vi "Final-MurphyE-Sub.vi"(0 "multimeter 1 in":refnum<visa-resource-name>, 1 "Measure? 2 Init Value":bool, 5 "multimeter 2 in":refnum<visa-resource-name>, 7 "function gen in":refnum<visa-resource-name>, 9 "n":i32, 11 "vp-pk to pk array of values":dbl[](array[numeric]), 12 "freq array input":dbl[](array[numeric])) -> (3 "Possible resonant f0 freq\nfor run 2":dbl, 4 "multimeter 1 out":refnum<visa-resource-name>, 6 "multimeter 2 out":refnum<visa-resource-name>, 8 "function gen out":refnum<visa-resource-name>, 10 "freq array output (used)":dbl[](array[numeric]), 13 "vr/vfg rms Cluster for graph":cluster{"freq run 1 list":dbl[], dbl[]}, 14 "Run 2 True Condition Measure Button":bool, 15 "vr/vfg array":dbl[](array[numeric]))   [LabVIEW 2018]
doc: "main while loop for labview program"
uses:
  <vilib>/Analysis/NI_AALBase.lvlib
panel:
  out "Ready For Next Step":bool
  in  "Auto Advance to Next":bool
  in  "Start Taking Measurements?":bool
  out "v across v0 2":dbl
  out "vrms Array":dbl[](array[numeric])
  in  "stop":bool
  out "# Measurements":i32
  out "# Runs":i32
  out "Desired VRMS  (V)":dbl=1.0 min=0.1 max=5.7 step=0.1
  out "freq":dbl
  out "vrms array perfect":dbl[](array[numeric])
  out "Vr0 Vrms":T1(graph)
  out "vfg":dbl
  out "vfg array":dbl[](array[numeric])
  out "Vfg Vrms":T1(graph)
  out "Transfer Function vr0/vfg Vrms":T1(graph)
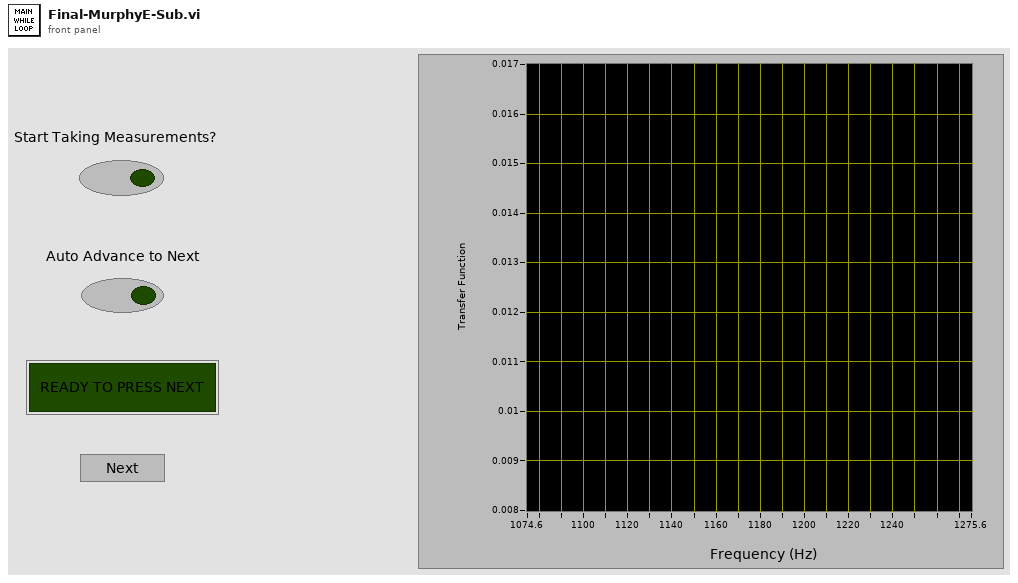
[diagram p1: front panel]
types:
  T1 = cluster{"Ramp Pattern":dbl[], "vrms array":dbl[]}
  T2 = cluster{"freq array input":dbl[], "measured vrms array":dbl[]}
  T3 = cluster{"freq array input":dbl[], "vrms across fg":dbl[]}
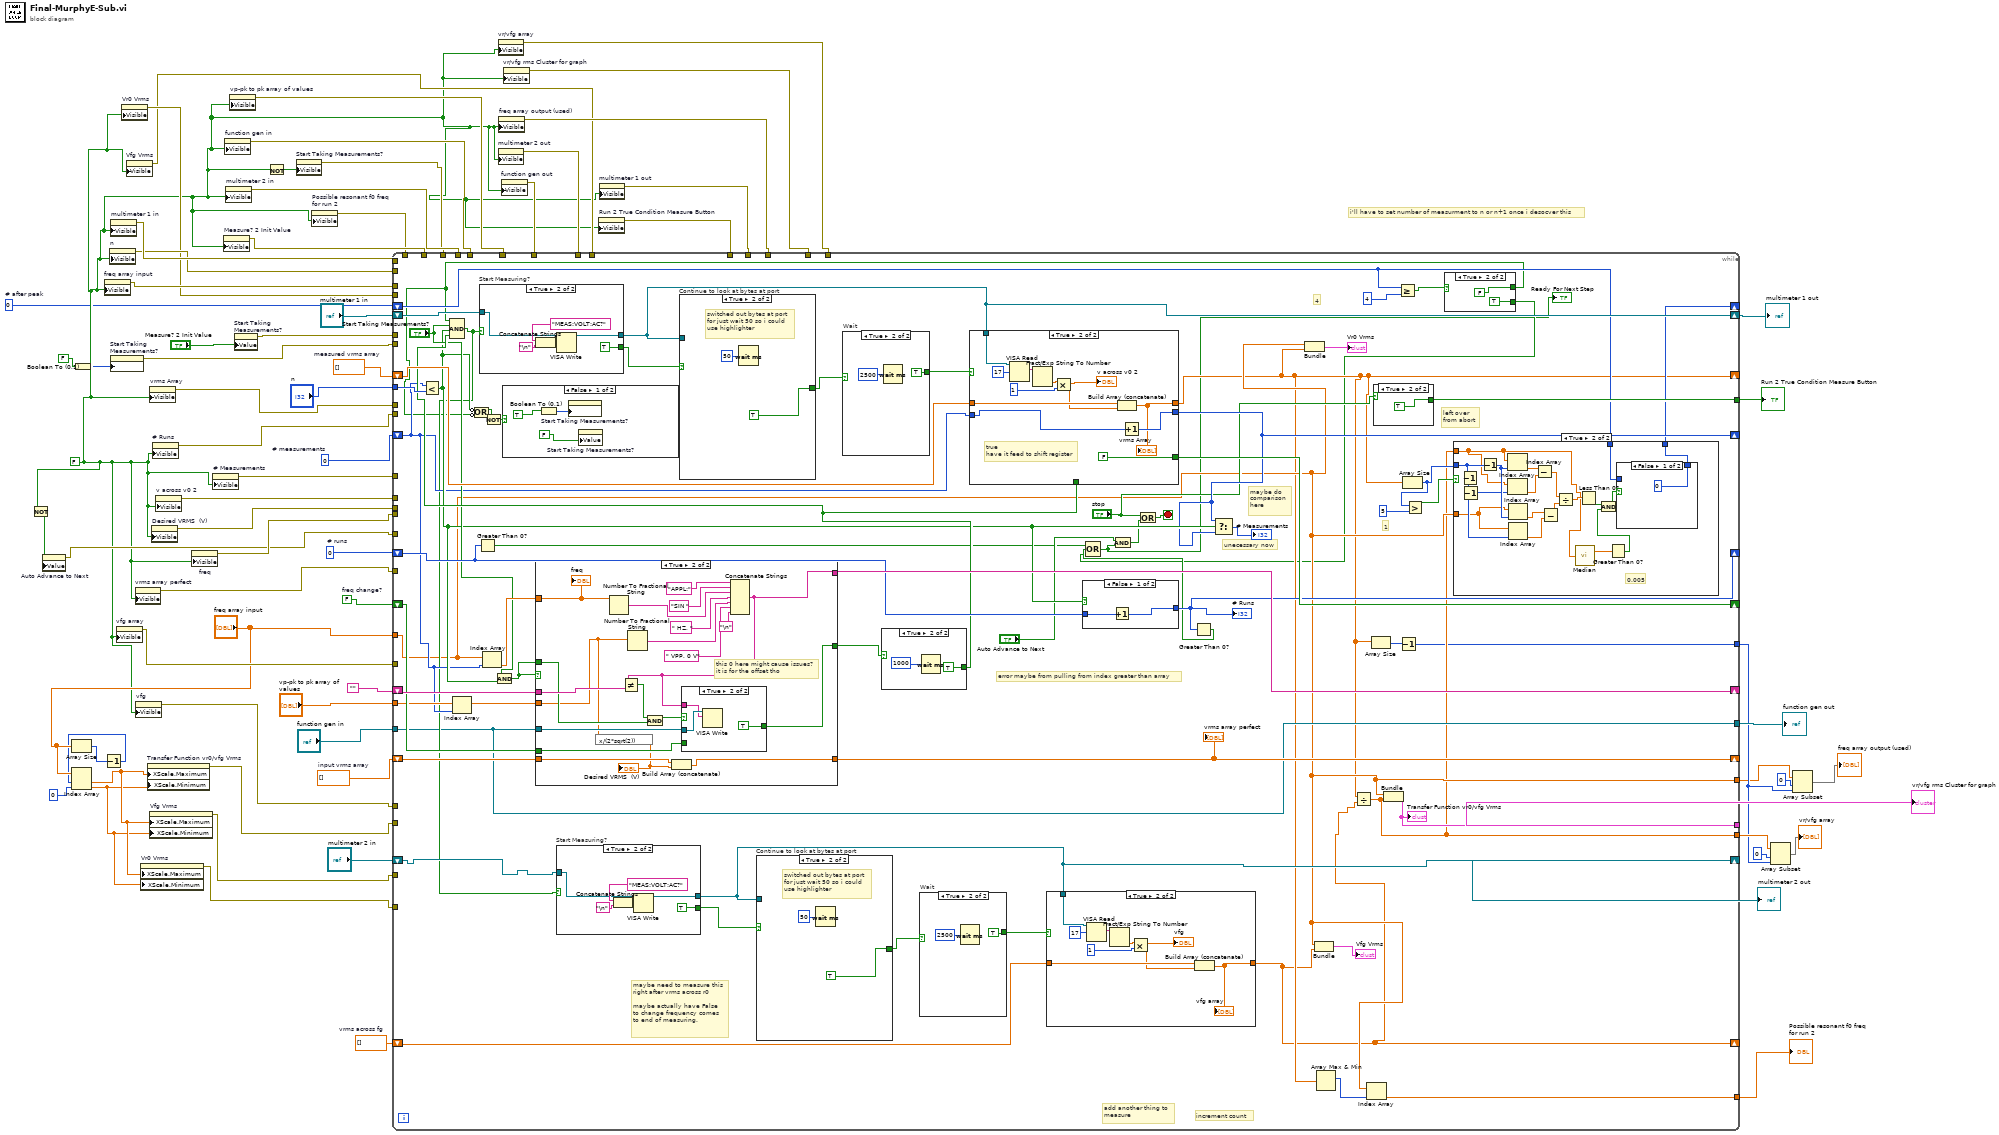
[diagram p0: block diagram]
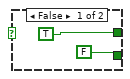
[diagram p2: hidden frame]
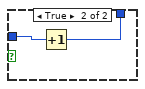
[diagram p4: hidden frame]
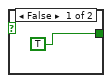
[diagram p5: hidden frame]
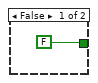
[diagram p7: hidden frame]
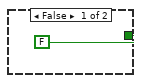
[diagram p8: hidden frame]
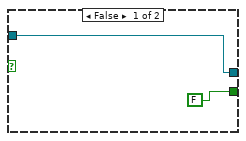
[diagram p9: hidden frame]
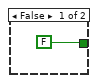
[diagram p16: hidden frame]
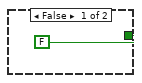
[diagram p17: hidden frame]
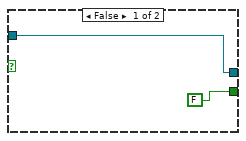
[diagram p18: hidden frame]
diagram:
  w9 = 0  # # after peak
  w68 = 0  # # measurements
  w13 = FALSE
  w60 = dbl[] []  # vrms across fg
  w62 = dbl[] []  # input vrms array
  w66 = FALSE  # freq change?
  w67 = 0  # # runs
  w70 = dbl[] []  # measured vrms array
  # "i'll have to set number of measurment to n or n+1 once i desocver this"
  n1 = Not(x=w13) -> (.not. x?=w8:bool)
  n2 = property on="Auto Advance to Next" class="Bool (strict)"("Value"=w8) -> (error out=w14:errorcluster)  [unwired: 2 in, 1 out]
  n3 = Array Size(array="freq array input") -> (size(s)=w43:i32)
  n4 = Boolean To (0,1)(Boolean=FALSE) -> (0, 1=w10:i16)
  n5 = property on="freq array input" class="Arr (strict)"("Visible"=w13) -> (error out=w20:errorcluster)  [unwired: 2 in, 1 out]
  n6 = Decrement(x=w43) -> (x-1=w42:i32)
  n7 = Index Array(array="freq array input", index #1=w42, index #2=0 ("index")) -> (element #1=w40:dbl, element #2=w39:dbl)
  n8 = property on="n" class="DigNum (strict)"("Visible"=w13) -> (error out=w21:errorcluster)  [unwired: 2 in, 1 out]
  n9 = property on="multimeter 1 in" class="VISAName"("Visible"=w13) -> (error out=w22:errorcluster)  [unwired: 2 in, 1 out]
  n10 = property on="Start Taking Measurements?" class="Bool (strict)"("DisabledEnum"=w10) -> (error out=w12:errorcluster)  [unwired: 2 in, 1 out]
  n11 = property on="vfg array" class="Arr (strict)"("Visible"=w13) -> (error out=w53:errorcluster)  [unwired: 2 in, 1 out]
  n12 = property on="Vr0 Vrms" class="XYGraph (strict)"("Visible"=w13) -> (error out=w16:errorcluster)  [unwired: 2 in, 1 out]
  n13 = property on="Vfg Vrms" class="XYGraph (strict)"("Visible"=w13) -> (error out=w15:errorcluster)  [unwired: 2 in, 1 out]
  n14 = property on="vrms array perfect" class="Arr (strict)"("Visible"=w13) -> (error out=w56:errorcluster)  [unwired: 2 in, 1 out]
  n15 = property on="vfg" class="DigNum (strict)"("Visible"=w13) -> (error out=w52:errorcluster)  [unwired: 2 in, 1 out]
  n16 = property on="Vr0 Vrms" class="XYGraph (strict)"("XScale.Maximum"=w40, "XScale.Minimum"=w39) -> (error out=w36:errorcluster)  [unwired: 2 in, 1 out]
  n17 = property on="Transfer Function vr0/vfg Vrms" class="XYGraph (strict)"("XScale.Maximum"=w40, "XScale.Minimum"=w39) -> (error out=w38:errorcluster)  [unwired: 2 in, 1 out]
  n18 = property on="vrms Array" class="Arr (strict)"("Visible"=w13) -> (error out=w54:errorcluster)  [unwired: 2 in, 1 out]
  n19 = property on="Vfg Vrms" class="XYGraph (strict)"("XScale.Maximum"=w40, "XScale.Minimum"=w39) -> (error out=w37:errorcluster)  [unwired: 2 in, 1 out]
  n20 = property on="Desired VRMS  (V)" class="DigNum (strict)"("Visible"=w13) -> (error out=w58:errorcluster)  [unwired: 2 in, 1 out]
  n21 = property on="# Runs" class="DigNum (strict)"("Visible"=w13) -> (error out=w55:errorcluster)  [unwired: 2 in, 1 out]
  n22 = property on="v across v0 2" class="DigNum (strict)"("Visible"=w13) -> (error out=w59:errorcluster)  [unwired: 2 in, 1 out]
  n23 = property on="freq" class="DigNum (strict)"("Visible"=w13) -> (error out=w57:errorcluster)  [unwired: 2 in, 1 out]
  n24 = property on="# Measurements" class="DigNum (strict)"("Visible"=w13) -> (error out=w45:errorcluster)  [unwired: 2 in, 1 out]
  n25 = property on="Measure? 2 Init Value" class="Bool (strict)"("Visible"=w13) -> (error out=w23:errorcluster)  [unwired: 2 in, 1 out]
  n26 = property on="function gen in" class="VISAName"("Visible"=w13) -> (error out=w25:errorcluster)  [unwired: 2 in, 1 out]
  n27 = property on="multimeter 2 in" class="VISAName"("Visible"=w13) -> (error out=w24:errorcluster)  [unwired: 2 in, 1 out]
  n28 = property on="vp-pk to pk array of values" class="Arr (strict)"("Visible"=w13) -> (error out=w26:errorcluster)  [unwired: 2 in, 1 out]
  n29 = property on="Start Taking Measurements?" class="Bool (strict)"("Value"="Measure? 2 Init Value") -> (error out=w35:errorcluster)  [unwired: 2 in, 1 out]
  n30 = Not(x=w13) -> (.not. x?=w17:bool)
  n31 = property on="Start Taking Measurements?" class="Bool (strict)"("Visible"=w17) -> (error out=w18:errorcluster)  [unwired: 2 in, 1 out]
  n32 = property on="Possible resonant f0 freq\nfor run 2" class="DigNum (strict)"("Visible"=w13) -> (error out=w19:errorcluster)  [unwired: 2 in, 1 out]
  n33 = property on="vr/vfg array" class="Arr (strict)"("Visible"=w13) -> (error out=w33:errorcluster)  [unwired: 2 in, 1 out]
  n34 = property on="multimeter 2 out" class="VISAName"("Visible"=w13) -> (error out=w27:errorcluster)  [unwired: 2 in, 1 out]
  n35 = property on="freq array output (used)" class="Arr (strict)"("Visible"=w13) -> (error out=w31:errorcluster)  [unwired: 2 in, 1 out]
  n36 = property on="function gen out" class="VISAName"("Visible"=w13) -> (error out=w28:errorcluster)  [unwired: 2 in, 1 out]
  n37 = property on="vr/vfg rms Cluster for graph" class="Clust (strict)"("Visible"=w13) -> (error out=w32:errorcluster)  [unwired: 2 in, 1 out]
  n38 = property on="Run 2 True Condition Measure Button" class="Bool (strict)"("Visible"=w13) -> (error out=w30:errorcluster)  [unwired: 2 in, 1 out]
  n39 = property on="multimeter 1 out" class="VISAName"("Visible"=w13) -> (error out=w29:errorcluster)  [unwired: 2 in, 1 out]
  n40 = while {
    shift-right: [w132] -> w46
    shift-left: "multimeter 1 in" -> [w131]
    shift-right: [w109] -> _
    shift-left: w68 -> [w113]
    shift-right: [w77] -> _
    shift-left: w70 -> [w130]
    tunnel: "n" -> [w129]
    shift-right: [w119] -> _
    shift-left: w67 -> [w122]
    tunnel: "freq array input" -> [w86]
    tunnel: "function gen in" -> [w99]
    shift-right: [w126] -> _
    shift-left: "" -> [w127]
    shift-right: [w123] -> _
    shift-left: w66 -> [w124]
    tunnel: "vp-pk to pk array of values" -> [w115]
    shift-right: [w111] -> _
    shift-left: w62 -> [w112]
    shift-right: [w104] -> w49
    shift-left: "multimeter 2 in" -> [w105]
    shift-right: [w75] -> _
    shift-left: w60 -> [w103]
    tunnel: [w99] -> w48
    tunnel: [w98] -> w47
    tunnel: [w97] -> w50
    tunnel: w59 -> [_]
    tunnel: w58 -> [_]
    tunnel: w57 -> [_]
    tunnel: w56 -> [_]
    tunnel: w55 -> [_]
    tunnel: w54 -> [_]
    tunnel: w53 -> [_]
    tunnel: w52 -> [_]
    tunnel: [w86] -> w2
    tunnel: [w85] -> w6
    tunnel: [w96] -> w51
    tunnel: w45 -> [_]
    tunnel: w38 -> [_]
    tunnel: w37 -> [_]
    tunnel: w36 -> [_]
    tunnel: w35 -> [_]
    tunnel: w33 -> [_]
    tunnel: w32 -> [_]
    tunnel: w31 -> [_]
    tunnel: w30 -> [_]
    tunnel: w29 -> [_]
    tunnel: w28 -> [_]
    tunnel: w27 -> [_]
    tunnel: w26 -> [_]
    tunnel: w25 -> [_]
    tunnel: w24 -> [_]
    tunnel: w23 -> [_]
    tunnel: w22 -> [_]
    tunnel: w21 -> [_]
    tunnel: w20 -> [_]
    tunnel: w19 -> [_]
    tunnel: w18 -> [_]
    tunnel: w16 -> [_]
    tunnel: w15 -> [_]
    tunnel: w14 -> [_]
    tunnel: w12 -> [_]
    shift-right: [w84] -> _
    shift-left: w9 -> [w83]
    tunnel: [w74] -> w4
    stop <- w95 stop-if-true
    # "1"
    # "4"
    # "increment count"
    # "add another thing to\nmeasure"
    # "left over\nfrom abort"
    # "maybe need to measure this\nright after vrms across r0\n\nmaybe actually have False\nto change frequency comes\nto end of measuring."
    # "unecessary now"
    # "maybe do\ncomparison\nhere"
    # "error maybe from pulling from index greater than array"
    n41 = Less?(x=w113, y=w129) -> (x < y?=w117:bool)
    n42 = Index Array(array=w115, index=w113) -> (element=w114:dbl)
    n43 = Greater Than 0?(x=w122) -> (x > 0?=w90:bool)
    n44 = Index Array(array=w86, index=w113) -> (element=w125:dbl)
    n45 = Compound Arithmetic op=AND("Start Taking Measurements?", w117) -> (w116:bool)
    n46 = case shown="True" w116 {
      tunnel: w99 -> [_ w205]
      tunnel: w127 -> [w193 w204]
      tunnel: [w193 w203] -> w126
      tunnel: w125 -> [_ w202]
      tunnel: w116 -> [_ w200]
      tunnel: w124 -> [w192 w199]
      tunnel: [w192 w198] -> w121
      tunnel: w114 -> [_ w197]
      tunnel: w112 -> [w191 w196]
      tunnel: [w191 w194] -> w111
      frame False {
      }
      frame True {
        # "this 0 here might cause issues?\nit is for the offset tho"
        n47 = expression code="x/(2*sqrt(2))"(w197) -> (w195:dbl)
        "Desired VRMS  (V)" <- w195
        n48 = Number To Fractional String(number=w202) -> (F-format string=w211:string)  [unwired: 3 in]
        n49 = Number To Fractional String(number=w197) -> (F-format string=w209:string)  [unwired: 3 in]
        n50 = Build Array (concatenate)(w196, w195) -> (w194:dbl[])
        n51 = Concatenate Strings("APPL:", "SIN ", w211, " HZ, ", w209, " VPP, 0 V", "\n") -> (w203:string)
        n52 = Not Equal?(x=w203, y=w204) -> (x != y?=w206:bool)
        n53 = Compound Arithmetic op=AND(w206, w200) -> (w201:bool)
        n54 = case shown="True" w201 {
          tunnel: w203 -> [_ w216]
          tunnel: w205 -> [_ w217]
          tunnel: [w214 TRUE] -> w198
          tunnel: w199 -> [w214 _]
          frame False {
          }
          frame True {
            n55 = VISA Write(VISA resource name=w217, write buffer=w216) -> ()  [unwired: 1 in, 3 out]
          }
        }
        "freq" <- w202
      }
    }
    "vrms array perfect" <- w111
    n56 = case shown="True" w121 {
      selector: w121 -> [w188 _]
      tunnel: [w188 TRUE] -> w120
      frame False {
      }
      frame True {
        n57 = Wait (ms)(milliseconds to wait=u32 1000) -> ()  [unwired: 1 out]
      }
    }
    n58 = case shown="False" w117 {
      tunnel: w122 -> [w219 w220]
      tunnel: [w218 w220] -> w119
      frame False {
        n59 = Increment(x=w219) -> (x+1=w218:i32)
      }
      frame True {
      }
    }
    "# Runs" <- w119
    n60 = Greater Than 0?(x=w119) -> (x > 0?=w93:bool)
    n61 = case shown="True" "stop" {
      tunnel: [TRUE TRUE] -> w98
      frame False {
      }
      frame True {
      }
    }
    n62 = Greater Or Equal?(x=w83, y=4) -> (x >= y?=w81:bool)
    n63 = case shown="True" w81 {
      tunnel: [TRUE FALSE] -> w79
      tunnel: [FALSE TRUE] -> w73
      frame False {
      }
      frame True {
      }
    }
    n64 = Compound Arithmetic op=AND(w79, "Start Taking Measurements?", w117, w120) -> (w102:bool)
    n65 = Compound Arithmetic op=OR(invert w117, invert w79) -> (w80:bool)
    n66 = case "Start Measuring?" shown="True" w102 {
      tunnel: [FALSE TRUE] -> w135
      tunnel: [w244 w247] -> w132
      tunnel: w131 -> [w244 w246]
      frame False {
      }
      frame True {
        n67 = Concatenate Strings("MEAS:VOLT:AC?", "\n") -> (w250:string)
        n68 = VISA Write(VISA resource name=w246, write buffer=w250) -> (VISA resource name out=w247:refnum<visa-resource-name>)  [unwired: 1 in, 2 out]
      }
    }
    n69 = Not(x=w80) -> (.not. x?=w78:bool)
    n70 = case shown="False" w78 {
      frame False {
        n71 = Boolean To (0,1)(Boolean=TRUE) -> (0, 1=w221:i16)
        n72 = property on="Start Taking Measurements?" class="Bool (strict)"("DisabledEnum"=w221) -> ()  [unwired: 2 in, 2 out]
        n73 = property on="Start Taking Measurements?" class="Bool (strict)"("Value"=FALSE) -> ()  [unwired: 2 in, 2 out]
      }
      frame True {
      }
    }
    n74 = case "Start Measuring?" shown="True" w102 {
      tunnel: [FALSE TRUE] -> w108
      tunnel: [w180 w183] -> w104
      tunnel: w105 -> [w180 w182]
      frame False {
      }
      frame True {
        n75 = Concatenate Strings("MEAS:VOLT:AC?", "\n") -> (w186:string)
        n76 = VISA Write(VISA resource name=w182, write buffer=w186) -> (VISA resource name out=w183:refnum<visa-resource-name>)  [unwired: 1 in, 2 out]
      }
    }
    n77 = case "Continue to look at bytes at port" shown="True" w135 {
      tunnel: w132 -> [_ _]
      tunnel: [FALSE TRUE] -> w134
      frame False {
      }
      frame True {
        # "switched out bytes at port\nfor just wait 50 so i could\nuse highlighter"
        n78 = Wait (ms)(milliseconds to wait=u32 50) -> ()  [unwired: 1 out]
      }
    }
    n79 = case "Continue to look at bytes at port" shown="True" w108 {
      tunnel: w104 -> [_ _]
      tunnel: [FALSE TRUE] -> w107
      frame False {
      }
      frame True {
        # "switched out bytes at port\nfor just wait 50 so i could\nuse highlighter"
        n80 = Wait (ms)(milliseconds to wait=u32 50) -> ()  [unwired: 1 out]
      }
    }
    n81 = case "Wait" shown="True" w134 {
      tunnel: [FALSE TRUE] -> w133
      frame False {
      }
      frame True {
        n82 = Wait (ms)(milliseconds to wait=u32 2500) -> ()  [unwired: 1 out]
      }
    }
    n83 = case "Wait" shown="True" w107 {
      tunnel: [FALSE TRUE] -> w106
      frame False {
      }
      frame True {
        n84 = Wait (ms)(milliseconds to wait=u32 2500) -> ()  [unwired: 1 out]
      }
    }
    n85 = case shown="True" w133 {
      tunnel: w132 -> [_ w233]
      tunnel: w113 -> [w226 w229]
      tunnel: [w226 w231] -> w109
      tunnel: w130 -> [w225 w232]
      tunnel: [w225 w230] -> w77
      tunnel: [w224 FALSE] -> w123
      tunnel: w120 -> [w224 _]
      frame False {
      }
      frame True {
        # "true\nhave it feed to shift register"
        n86 = VISA Read(VISA resource name=w233, byte count=17) -> (read buffer=w237:string)  [unwired: 1 in, 3 out]
        n87 = Fract/Exp String To Number(string=w237) -> (number=w234:dbl)  [unwired: 3 in, 1 out]
        n88 = Multiply(x=w234, y=1) -> (x*y=w227:dbl)
        "v across v0 2" <- w227
        n89 = Build Array (concatenate)(w232, w227) -> (w230:dbl[])
        "vrms Array" <- w230
        n90 = Increment(x=w229) -> (x+1=w231:i32)
      }
    }
    n91 = case shown="True" w106 {
      tunnel: w104 -> [_ w169]
      tunnel: w103 -> [w165 w168]
      tunnel: [w165 w166] -> w75
      frame False {
      }
      frame True {
        n92 = VISA Read(VISA resource name=w169, byte count=17) -> (read buffer=w173:string)  [unwired: 1 in, 3 out]
        n93 = Fract/Exp String To Number(string=w173) -> (number=w170:dbl)  [unwired: 3 in, 1 out]
        n94 = Multiply(x=w170, y=1) -> (x*y=w167:dbl)
        "vfg" <- w167
        n95 = Build Array (concatenate)(w168, w167) -> (w166:dbl[])
        "vfg array" <- w166
      }
    }
    n96 = Compound Arithmetic op=OR(w90, w93, w73) -> (w72:bool)
    "Ready For Next Step" <- w72
    n97 = And(x="Auto Advance to Next", y=w72) -> (x .and. y?=w91:bool)
    n98 = Compound Arithmetic op=OR("stop", w91) -> (w95:bool)
    n99 = Select(t=w109, s=w117, f=w109) -> (s? t:f=→"# Measurements":i32)
    n100 = Bundle("freq array input"=w86, "measured vrms array"=w77) -> (→"Vr0 Vrms":T2)  [unwired: 1 in]
    n101 = Bundle("freq array input"=w86, "vrms across fg"=w75) -> (→"Vfg Vrms":T3)  [unwired: 1 in]
    n102 = Array Max & Min(array=w77) -> (max index (indices)=w100:i32)  [unwired: 3 out]
    n103 = Divide(x=w77, y=w75) -> (x/y=w85:dbl[])
    n104 = Index Array(array=w86, index=w100) -> (element=w97:dbl)
    n105 = Array Size(array=w77) -> (size(s)=w76:i32)
    n106 = Bundle("freq array input"=w86, w85) -> (w96:cluster{"freq array input":dbl[], dbl[]})  [unwired: 1 in]
    "Transfer Function vr0/vfg Vrms" <- w96
    n107 = Decrement(x=w76) -> (x-1=w74:i32)
    n108 = Array Size(array=w77) -> (size(s)=w87:i32)
    n109 = Greater?(x=w87, y=5) -> (0:w88:bool)
    n110 = case shown="True" w88 {
      tunnel: w87 -> [_ w159]
      tunnel: w85 -> [_ w145]
      tunnel: w86 -> [_ w151]
      tunnel: w83 -> [w140 w147]
      tunnel: [w140 w146] -> w84
      frame False {
      }
      frame True {
        # "0.005"
        n111 = Decrement(x=w159) -> (x-1=w157:i32)
        n112 = Decrement(x=w157) -> (x-1=w156:i32)
        n113 = Decrement(x=w159) -> (x-1=w158:i32)
        n114 = Index Array(array=w145, index=w158) -> (element=w155:dbl)
        n115 = Index Array(array=w145, index=w156) -> (element=w154:dbl)
        n116 = Index Array(array=w151, index=w158) -> (element=w150:dbl)
        n117 = Index Array(array=w151, index=w156) -> (element=w149:dbl)
        n118 = Subtract(x=w155, y=w154) -> (x-y=w153:dbl)
        n119 = Subtract(x=w150, y=w149) -> (x-y=w148:dbl)
        n120 = Divide(x=w153, y=w148) -> (x/y=w152:dbl)
        n121 = call <vilib>:"Median.vi"("X"=w145) -> ("median"=w144:dbl)  [unwired: 1 out]
        n122 = Less Than 0?(x=w152) -> (x < 0?=w142:bool)
        n123 = Greater Than 0?(x=w144) -> (x > 0?=w141:bool)
        n124 = Compound Arithmetic op=AND(w142, w141) -> (w143:bool)
        n125 = case shown="False" w143 {
          tunnel: w147 -> [_ w162]
          tunnel: [0 w161] -> w146
          frame False {
          }
          frame True {
            n126 = Increment(x=w162) -> (x+1=w161:i32)
          }
        }
      }
    }
  }
  "vr/vfg rms Cluster for graph" <- w51
  "Possible resonant f0 freq\nfor run 2" <- w50
  "multimeter 2 out" <- w49
  "function gen out" <- w48
  "Run 2 True Condition Measure Button" <- w47
  "multimeter 1 out" <- w46
  n127 = Array Subset(array=w6, index=0, length=w4) -> (→"vr/vfg array":dbl[])
  n128 = Array Subset(array=w2, index=0, length=w4) -> (→"freq array output (used)":dbl[])
